vi "Serial Write.vi"(8 "error in (no error)":errorcluster, 9 "timeout (ms)":i32, 10 "data":u8[](array[numeric]), 11 "VISA resource":refnum<visa-resource-name>) -> (0 "error out":errorcluster, 1 "timed out?":bool)   [LabVIEW 2018, in "SubVIs.lvlib" / "Serial Shared Components.lvlib"]
doc: "Performs a write on the serial port."
uses:
  Serial Shared Components.lvlib
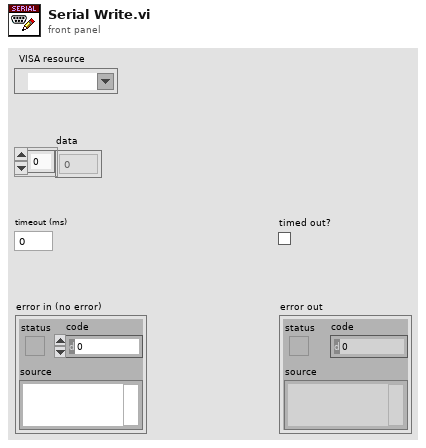
[diagram p1: front panel]
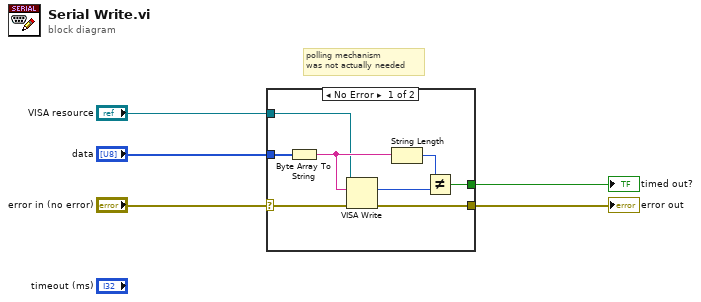
[diagram p0: block diagram]
diagram:
  # "polling mechanism\nwas not actually needed"
  n1 = case shown="No Error" "error in (no error)" {
    selector: "error in (no error)" -> [w6 w14]
    tunnel: "data" -> [w13 _]
    tunnel: [w9 _] -> w2
    tunnel: [w8 w14] -> w4
    tunnel: "VISA resource" -> [w7 _]
    frame No Error {
      n2 = Byte Array To String(unsigned byte array=w13) -> (string=w12:string)
      n3 = VISA Write(VISA resource name=w7, write buffer=w12, error in (no error)=w6) -> (return count=w11:u32, error out=w8:errorcluster)  [unwired: 1 out]
      n4 = String Length(string=w12) -> (length=w10:i32)
      n5 = Not Equal?(x=w10, y=w11) -> (x != y?=w9:bool)
    }
    frame Error {
    }
  }
  "timed out?" <- w2
  "error out" <- w4
